vi "compute_linear_regression.vi"(0 "chemin du fichier":path) -> (1 "Best AL capteur 1":dbl[](array[numeric]), 2 "Best AL capteur 2":dbl[](array[numeric]), 3 "Best AL capteur 3":dbl[](array[numeric]), 4 "Best AL capteur 4":dbl[](array[numeric]))   [LabVIEW 2020]
panel:
  out "capteur 4 Graph":cluster{i32[], "Best Linear Fit":dbl[]}[](graph)
  out "capteur 3 Graph":cluster{i32[], "Best Linear Fit":dbl[]}[](graph)
  out "Capteur 2 Graph":cluster{i32[], "Y":dbl[]}[](graph)
  out "Capteur 1 Graph":cluster{i32[], "Best Linear Fit":dbl[]}[](graph)
  out "pente capteur 4":dbl
  out "pente capteur 3":dbl
  out "pente capteur 2":dbl
  out "pente capteur 1":dbl
  # "À Partir du fichier de mésures, nous effectuons un ajustement de linéaire sur\n  les différentes valeurs relévées par chaque capteur, Puis nous recupérons la pente et le meilleur\n  ajustement linéaire correpondant.\n   X = tableau de mesures\n   Y = aX + b : droite de regression ==> Y contiendra le meilleur ajustement\n   a : pente\n   b :  coordonnée verticale de l'intersection entre la droite de régression Y et l'axe oX \n\n  === > NB: ENTRER LE CHEMIN DU FICHIER AVANT DE LANCER CE PROGRAMME <====="
  # "Graphes des ajustements linéaires obtenus après traitement"
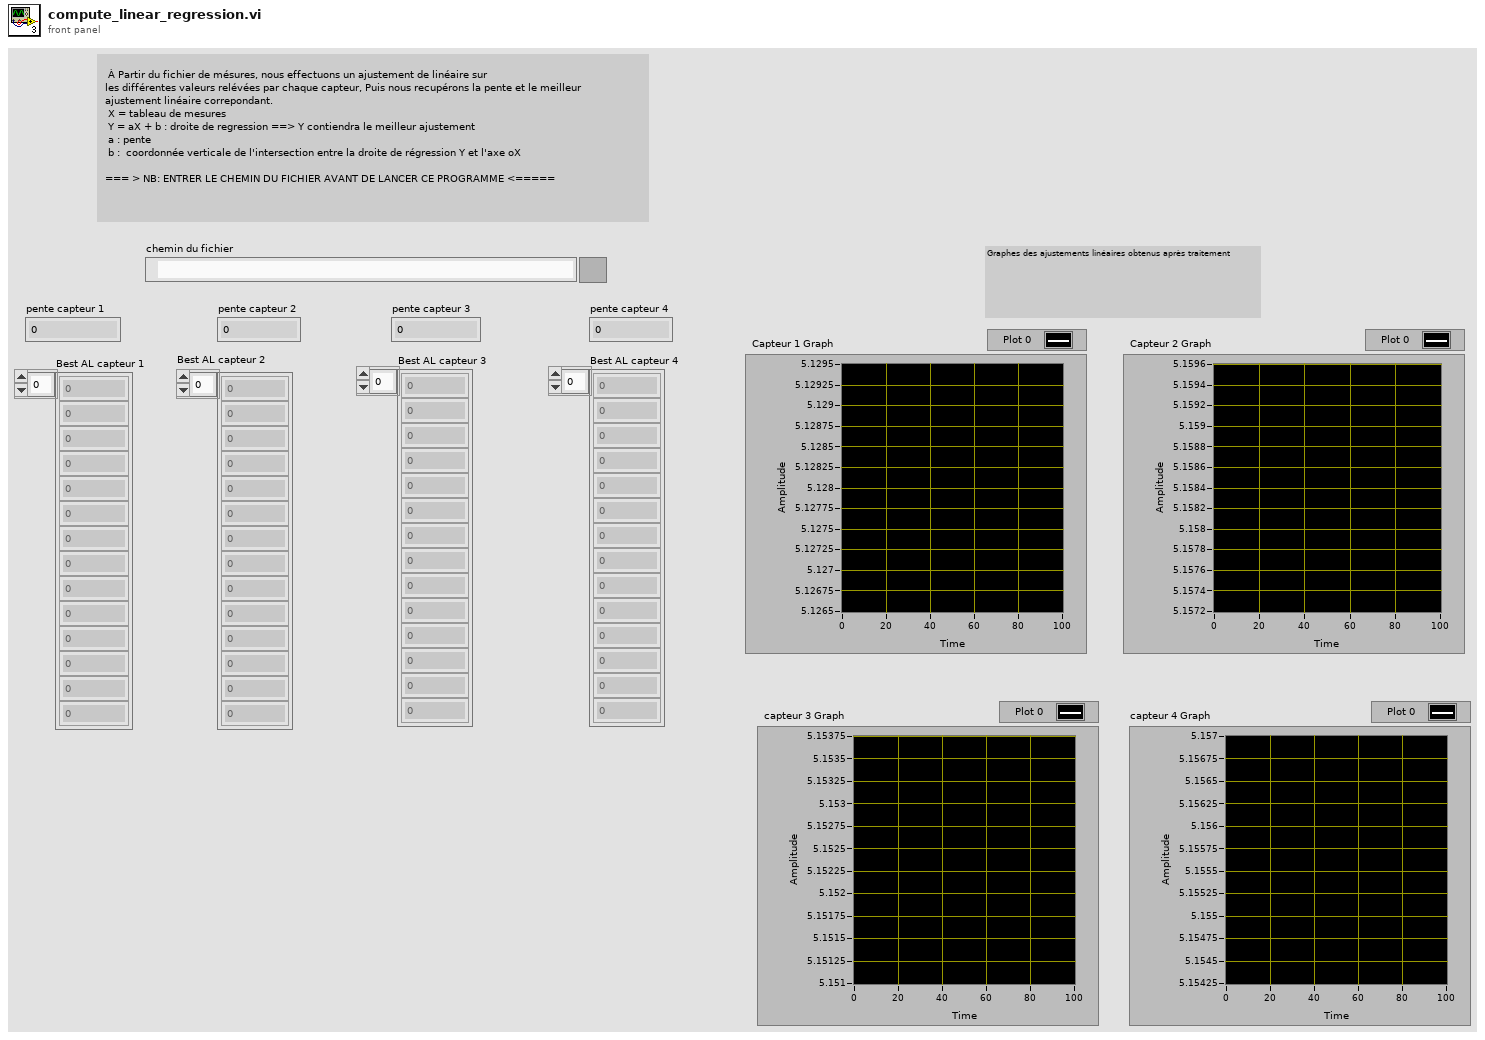
[diagram p1: front panel]
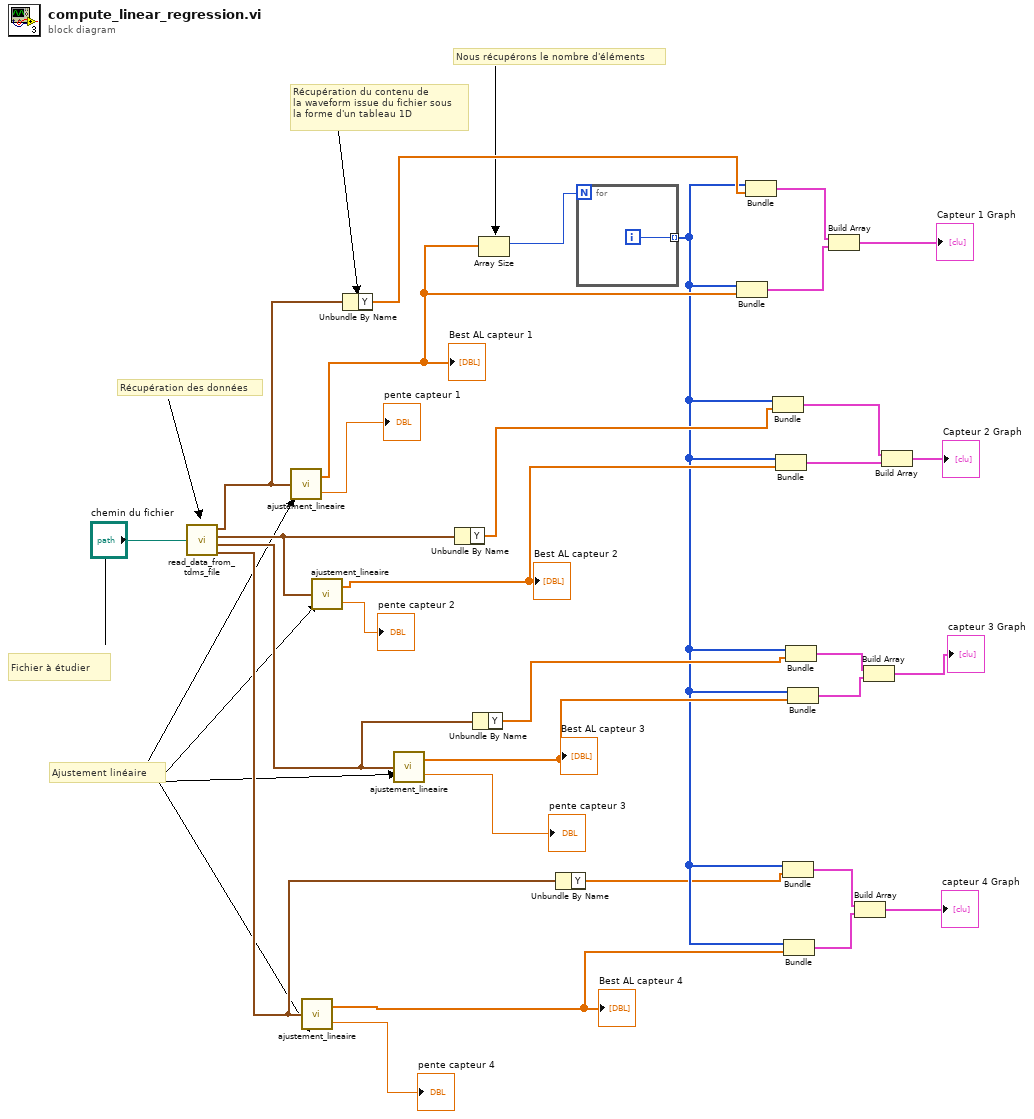
[diagram p0: block diagram]
diagram:
  # "Récupération du contenu de\nla waveform issue du fichier sous\nla forme d'un tableau 1D"
  # "Nous récupérons le nombre d'éléments"
  # "Ajustement linéaire"
  # "Récupération des données"
  # "Fichier à étudier"
  n1 = call "read_data_from_tdms_file.vi"("chemin du fichier"="chemin du fichier") -> ("capteur1"=w26:waveform(dbl), "capteur2"=w16:waveform(dbl), "capteur3"=w12:waveform(dbl), "capteur4"=w2:waveform(dbl))
  n2 = call "ajustement_lineaire.vi"("Y"=w26) -> ("Best Linear Fit"=w24:dbl[], "slope"=→"pente capteur 1":dbl)
  "Best AL capteur 1" <- w24
  n3 = call "ajustement_lineaire.vi"("Y"=w2) -> ("Best Linear Fit"=w3:dbl[], "slope"=→"pente capteur 4":dbl)
  "Best AL capteur 4" <- w3
  n4 = call "ajustement_lineaire.vi"("Y"=w16) -> ("Best Linear Fit"=w14:dbl[], "slope"=→"pente capteur 2":dbl)
  "Best AL capteur 2" <- w14
  n5 = Unbundle By Name(w26) -> ("Y"=w23:dbl[])
  n6 = call "ajustement_lineaire.vi"("Y"=w12) -> ("Best Linear Fit"=w13:dbl[], "slope"=→"pente capteur 3":dbl)
  "Best AL capteur 3" <- w13
  n7 = Unbundle By Name(w16) -> ("Y"=w15:dbl[])
  n8 = Unbundle By Name(w12) -> ("Y"=w11:dbl[])
  n9 = Array Size(array=w24) -> (size(s)=w25:i32)
  n10 = Unbundle By Name(w2) -> ("Y"=w1:dbl[])
  n11 = for {
    N: w25 -> [_]
    tunnel: [w32] -> w4 mode=indexing
    i -> [w32]
  }
  n12 = Bundle(w4, "Best Linear Fit"=w24) -> (w21:cluster{i32[], "Best Linear Fit":dbl[]})  [unwired: 1 in]
  n13 = Bundle(w4, "Y"=w23) -> (w22:cluster{i32[], "Y":dbl[]})  [unwired: 1 in]
  n14 = Bundle(w4, "Y"=w15) -> (w18:cluster{i32[], "Y":dbl[]})  [unwired: 1 in]
  n15 = Bundle(w4, "Best Linear Fit"=w14) -> (w19:cluster{i32[], "Best Linear Fit":dbl[]})  [unwired: 1 in]
  n16 = Bundle(w4, "Y"=w1) -> (w7:cluster{i32[], "Y":dbl[]})  [unwired: 1 in]
  n17 = Bundle(w4, "Best Linear Fit"=w3) -> (w6:cluster{i32[], "Best Linear Fit":dbl[]})  [unwired: 1 in]
  n18 = Bundle(w4, "Y"=w11) -> (w10:cluster{i32[], "Y":dbl[]})  [unwired: 1 in]
  n19 = Bundle(w4, "Best Linear Fit"=w13) -> (w9:cluster{i32[], "Best Linear Fit":dbl[]})  [unwired: 1 in]
  n20 = Build Array(w22, w21) -> (→"Capteur 1 Graph":cluster{i32[], "Best Linear Fit":dbl[]}[])
  n21 = Build Array(w7, w6) -> (→"capteur 4 Graph":cluster{i32[], "Best Linear Fit":dbl[]}[])
  n22 = Build Array(w10, w9) -> (→"capteur 3 Graph":cluster{i32[], "Best Linear Fit":dbl[]}[])
  n23 = Build Array(w18, w19) -> (→"Capteur 2 Graph":cluster{i32[], "Best Linear Fit":dbl[]}[])
